vi "ScanRobotMode.vi"(11 "robotMode in":string) -> (3 "robotMode out":T1)   [LabVIEW 2016, in "Universal Robot.lvclass"]
uses:
  Universal Robot.lvclass
  RobotMode.ctl
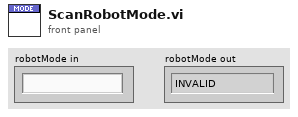
[diagram p1: front panel]
types:
  T1 = typedef "Universal Robot.lvclass/RobotMode.ctl" = enum16{"INVALID", "NO_CONTROLLER", "DISCONNECTED", "CONFIRM_SAFETY", "BOOTING", "POWER_OFF", "POWER_ON", "IDLE", "BACKDRIVE", "RUNNING"}
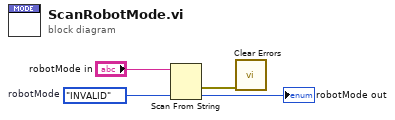
[diagram p0: block diagram]
diagram:
  w2 = RobotMode."INVALID"  # robotMode
  n1 = Scan From String(input string="robotMode in", default 1=w2) -> (error out=w1:errorcluster, output 1=→"robotMode out":T1)  [unwired: 3 in, 2 out]
  n2 = call <vilib>:"Clear Errors.vi"("error in (no error)"=w1) -> ()  [unwired: 5 in, 2 out]
